vi "Begin.vi"(8 "error in":errorcluster) -> (0 "error out":errorcluster)   [LabVIEW 2015]
doc: "Called before other user functions, this VI is expected to open initial I/O refnums, load in file data, and do all program initialization. Notice that the <B>error out</B> terminal is simply used for data flow. Wiring it to other structures or subVIs ensures that this VI runs first."
uses:
  <vilib>/Rock Robotics/WPI/DriverStation/WPI_DriverStationRobotMode2.ctl
  <vilib>/Rock Robotics/WPI/Joystick/WPI_JoystickDeviceEnum.ctl
  <vilib>/Rock Robotics/SystemInterfaces/DIO/FPGA_DIOPWMChannel.ctl
  <vilib>/Rock Robotics/SystemInterfaces/DIO/FPGA_DIOChannel.ctl
  <vilib>/Rock Robotics/WPI/Solenoid/WPI_SolenoidChannel.ctl
  <vilib>/Rock Robotics/SystemInterfaces/DIO/FPGA_DIORelayChannel.ctl
  <vilib>/Rock Robotics/WPI/Relay/WPI_RelayDirection.ctl
  Robot Global Data.vi
  <vilib>/Rock Robotics/Network Tables/NT Write String Array.vi
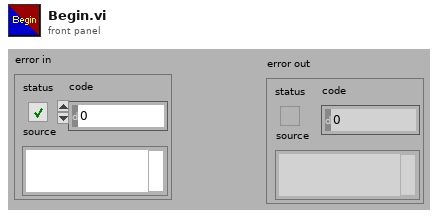
[diagram p1: front panel]
types:
  T1 = typedef "WPI_RelayDirection.ctl" = enum16{"Both directions", "Forward only", "Reverse only"}
  T2 = typedef "FPGA_DIORelayChannel.ctl" = enum8{"Relay 0", "Relay 1", "Relay 2", "Relay 3", "Invalid"}
  T3 = typedef "FPGA_DIOChannel.ctl" = enum8{"DIO 0", "DIO 1", "DIO 2", "DIO 3", "DIO 4", "DIO 5", "DIO 6", "DIO 7", "DIO 8", "DIO 9", "DIO MXP 0", "DIO MXP 1", "DIO MXP 2", "DIO MXP 3", "DIO MXP 4", "DIO MXP 5", "DIO MXP 6", "DIO MXP 7", "DIO MXP 8", "DIO MXP 9", "DIO MXP 10", "DIO MXP 11", "DIO MXP 12", "DIO MXP 13", "DIO MXP 14", "DIO MXP 15", "Invalid"}
  T4 = typedef "WPI_SolenoidChannel.ctl" = enum8{"Solenoid 0", "Solenoid 1", "Solenoid 2", "Solenoid 3", "Solenoid 4", "Solenoid 5", "Solenoid 6", "Solenoid 7", "Invalid"}
  T5 = typedef "FPGA_DIOPWMChannel.ctl" = enum8{"PWM 0", "PWM 1", "PWM 2", "PWM 3", "PWM 4", "PWM 5", "PWM 6", "PWM 7", "PWM 8", "PWM 9", "PWM MXP 0", "PWM MXP 1", "PWM MXP 2", "PWM MXP 3", "PWM MXP 4", "PWM MXP 5", "PWM MXP 6", "PWM MXP 7", "PWM MXP 8", "PWM MXP 9", "Invalid"}
  T6 = typedef "WPI_JoystickDeviceEnum.ctl" = enum16{"USB 0", "USB 1", "USB 2", "USB 3", "USB 4", "USB 5"}
  T7 = typedef "WPI_DriverStationRobotMode2.ctl" = enum16{"Autonomous Disabled", "Autonomous Enabled", "Teleop Disabled", "Teleop Enabled", "Disconnected", "Finish", "Test Disabled", "Test Enabled", "Emergency Stopped"}
  T8 = typedef "WPI_JoystickDevRef.ctl" = cluster{"Device":T6}
  T9 = typedef "WPI_RelayDevRef.ctl" = cluster{"DevStatus":errorcluster, "Relay Channel":T2, "Relay Direction":T1}
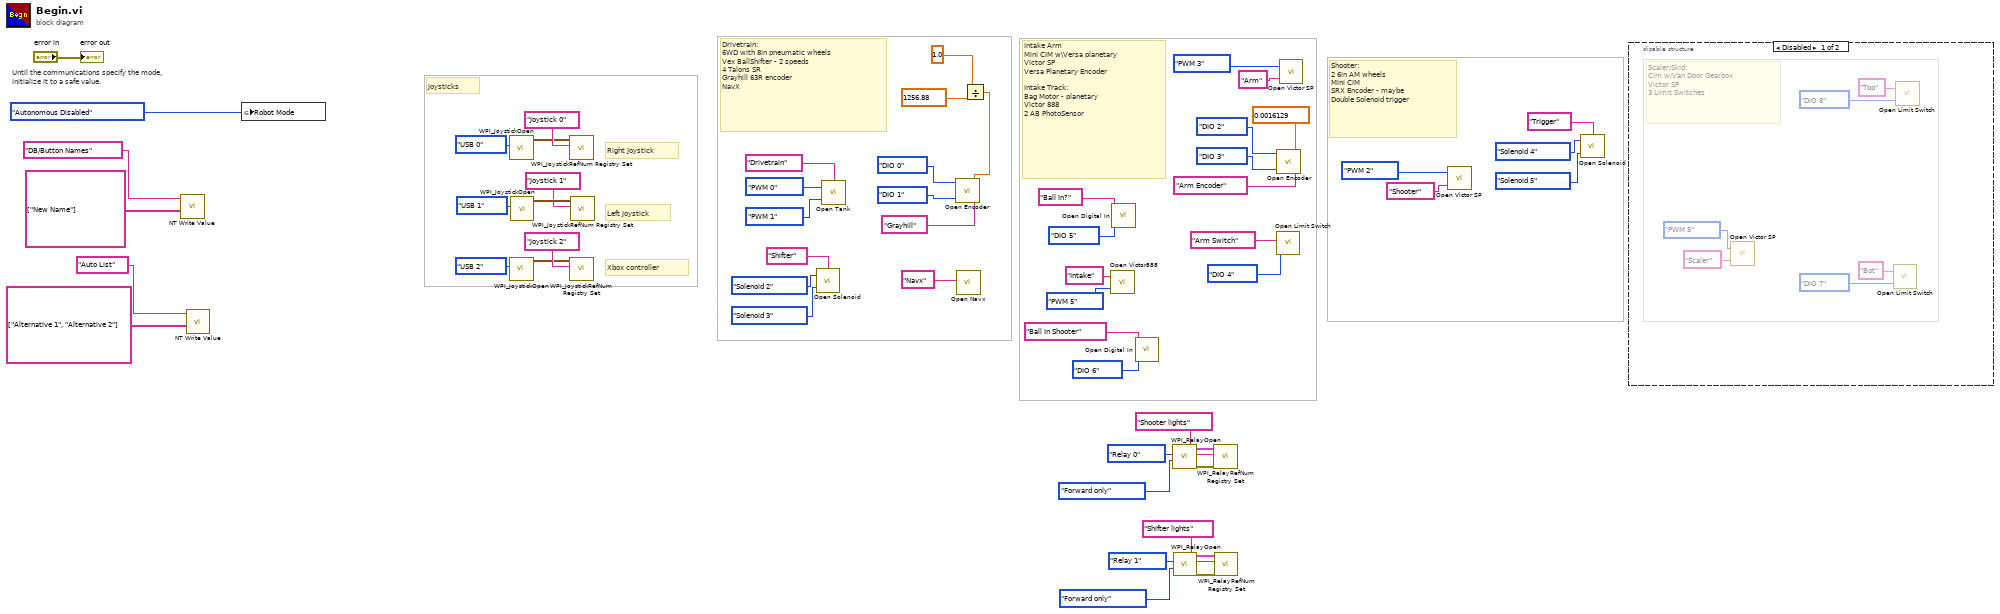
[diagram p0: block diagram]
diagram:
  # "Shooter:\n2 6in AM wheels\nMini CIM \nSRX Encoder - maybe\nDouble Solenoid trigger"
  # "Intake Arm\nMini CIM w\\Versa planetary\nVictor SP\nVersa Planetary Encoder\n\nIntake Track:\nBag Motor - planetary\nVictor 888\n2 AB PhotoSensor"
  # "Joysticks"
  # "Drivetrain:\n6WD with 8in pneumatic wheels\nVex BallShifter - 2 speeds\n4 Talons SR\nGrayhill 63R encoder\nNavX"
  # "Xbox controller"
  # "Left Joystick"
  # "Right Joystick"
  # "Until the communications specify the mode,\ninitialize it to a safe value."
  n1 = call-poly <vilib>:"NT Write Value.vi"("String Array"=string[] ["New Name"], "Name"="DB/Button Names") -> ()  [unwired: 9 in, 1 out]
  n2 = call-poly <vilib>:"NT Write Value.vi"("String Array"=string[] ["Alternative 1", "Alternative 2"], "Name"="Auto List") -> ()  [unwired: 9 in, 1 out]
  n3 = global write "Robot Global Data.vi" "Robot Mode"(WPI_DriverStationRobotMode2."Autonomous Disabled" ("Robot Mode")) -> ()
  n4 = call <vilib>:"WPI_JoystickOpen.vi"("JoystickDevice"=WPI_JoystickDeviceEnum."USB 0") -> ("JoystickDevRef"=w50:T8)  [unwired: 10 in]
  n5 = call <vilib>:"WPI_JoystickOpen.vi"("JoystickDevice"=WPI_JoystickDeviceEnum."USB 2") -> ("JoystickDevRef"=w44:T8)  [unwired: 10 in]
  n6 = call <vilib>:"WPI_JoystickOpen.vi"("JoystickDevice"=WPI_JoystickDeviceEnum."USB 1") -> ("JoystickDevRef"=w47:T8)  [unwired: 10 in]
  n7 = call <vilib>:"WPI_JoystickRefNum Registry Set.vi"("refnum name"="Joystick 0", "JoystickDevRef"=w50) -> ()  [unwired: 8 in, 2 out]
  n8 = call <vilib>:"WPI_JoystickRefNum Registry Set.vi"("refnum name"="Joystick 2", "JoystickDevRef"=w44) -> ()  [unwired: 8 in, 2 out]
  n9 = call <vilib>:"WPI_JoystickRefNum Registry Set.vi"("refnum name"="Joystick 1", "JoystickDevRef"=w47) -> ()  [unwired: 8 in, 2 out]
  n10 = call "Open Solenoid.vi"("refnum name"="Shifter", "Reverse Solenoid Channel"=WPI_SolenoidChannel."Solenoid 3", "Forward Solenoid Channel"=WPI_SolenoidChannel."Solenoid 2") -> ()  [unwired: 1 in]
  n11 = call "Open Tank.vi"("refnum name"="Drivetrain", "Right Motor"=FPGA_DIOPWMChannel."PWM 1", "Left Motor"=FPGA_DIOPWMChannel."PWM 0") -> ()  [unwired: 1 in]
  n12 = call "Open Navx.vi"("refnum name"="Navx") -> ()
  n13 = Divide(x=1.0, y=1256.88 ("DistancePerCount")) -> (x/y=w11:dbl)
  n14 = call "Open Encoder.vi"("refnum name"="Grayhill", "DistancePerCount"=w11, "B Channel"=FPGA_DIOChannel."DIO 1", "A Channel"=FPGA_DIOChannel."DIO 0") -> ()  [unwired: 1 in]
  n15 = call "Open Victor888.vi"("PWM Channel"=FPGA_DIOPWMChannel."PWM 5", "refnum name"="Intake") -> ()  [unwired: 2 in]
  n16 = call "Open Digital In.vi"("refnum name"="Ball In?", "DIO Channel"=FPGA_DIOChannel."DIO 5") -> ()  [unwired: 10 in]
  n17 = call "Open Digital In.vi"("refnum name"="Ball In Shooter", "DIO Channel"=FPGA_DIOChannel."DIO 6") -> ()  [unwired: 10 in]
  n18 = call <vilib>:"WPI_RelayOpen.vi"("Relay Direction"=WPI_RelayDirection."Forward only", "Relay Channel"=FPGA_DIORelayChannel."Relay 0") -> ("error out"=w10:errorcluster, "RelayDevRef"=w9:T9)  [unwired: 8 in]
  n19 = call <vilib>:"WPI_RelayOpen.vi"("Relay Direction"=WPI_RelayDirection."Forward only", "Relay Channel"=FPGA_DIORelayChannel."Relay 1") -> ("error out"=w1:errorcluster, "RelayDevRef"=w2:T9)  [unwired: 8 in]
  n20 = call <vilib>:"WPI_RelayRefNum Registry Set.vi"("error in (no error)"=w10, "refnum name"="Shooter lights", "RelayDevRef"=w9) -> ()  [unwired: 7 in, 2 out]
  n21 = call <vilib>:"WPI_RelayRefNum Registry Set.vi"("error in (no error)"=w1, "refnum name"="Shifter lights", "RelayDevRef"=w2) -> ()  [unwired: 7 in, 2 out]
  n22 = call "Open Limit Switch.vi"("DIO Channel"=FPGA_DIOChannel."DIO 4", "refnum name"="Arm Switch") -> ()  [unwired: 2 in]
  n23 = call "Open Encoder.vi"("refnum name"="Arm Encoder", "DistancePerCount"=0.0016129, "B Channel"=FPGA_DIOChannel."DIO 3", "A Channel"=FPGA_DIOChannel."DIO 2") -> ()  [unwired: 1 in]
  n24 = call "Open Victor SP.vi"("refnum name"="Arm", "PWM Channel"=FPGA_DIOPWMChannel."PWM 3") -> ()  [unwired: 1 in]
  n25 = call "Open Victor SP.vi"("refnum name"="Shooter", "PWM Channel"=FPGA_DIOPWMChannel."PWM 2") -> ()  [unwired: 1 in]
  n26 = call "Open Solenoid.vi"("refnum name"="Trigger", "Reverse Solenoid Channel"=WPI_SolenoidChannel."Solenoid 5", "Forward Solenoid Channel"=WPI_SolenoidChannel."Solenoid 4") -> ()  [unwired: 1 in]
  n27 = disable-structure shown="Disabled" {
    frame Disabled {
      # "Scaler/Skid:\nCim w/Van Door Gearbox\nVictor SP\n3 Limit Switches"
      n28 = call "Open Victor SP.vi"("refnum name"="Scaler", "PWM Channel"=FPGA_DIOPWMChannel."PWM 5") -> ()  [unwired: 1 in]
      n29 = call "Open Limit Switch.vi"("DIO Channel"=FPGA_DIOChannel."DIO 7", "refnum name"="Bot") -> ()  [unwired: 2 in]
      n30 = call "Open Limit Switch.vi"("DIO Channel"=FPGA_DIOChannel."DIO 8", "refnum name"="Top") -> ()  [unwired: 2 in]
    }
    frame Enabled {
    }
  }
  "error out" <- "error in"
